vi "ExCircularBufBin2x.vi"() -> ()   [LabVIEW 2010]
panel:
  in  "Software Accumulation":u32=1 min=1 step=1
  in  "Intensifier":bool
  in  "Temperature":dbl=-10.0 format="%.2f"
  in  "Exposure":dbl min=0.0 step=1e-06 format="%.5f"
  in  "stop":bool
  in  "Store":bool
  out "error out":errorcluster
  in  "error in (no error)":errorcluster
  # "ExCircularBufBin2x:\nThis example only works with cameras with circualar buffer capability. This routine will continously display an image binned by 2 in both the x and the y direction. It will store in append mode the frames while the store toggle switch is on."
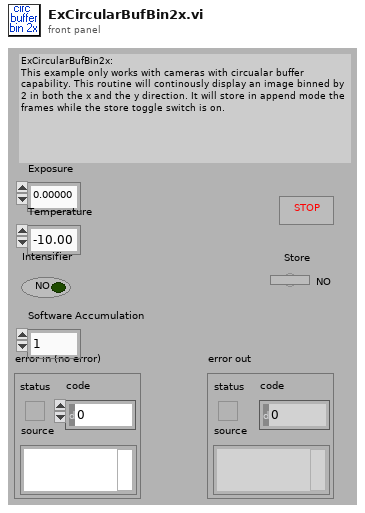
[diagram p1: front panel]
types:
  T1 = cluster{"acquire focus mode":u32, "Exposure":dbl, "Number of Images":u32, "Software Accumulation":u32}
  T2 = cluster{"Camera Handle":u32, "Pulser Handle":u32, "File Handle":u32, "Display Handle":u32, "Image Handle":u32}
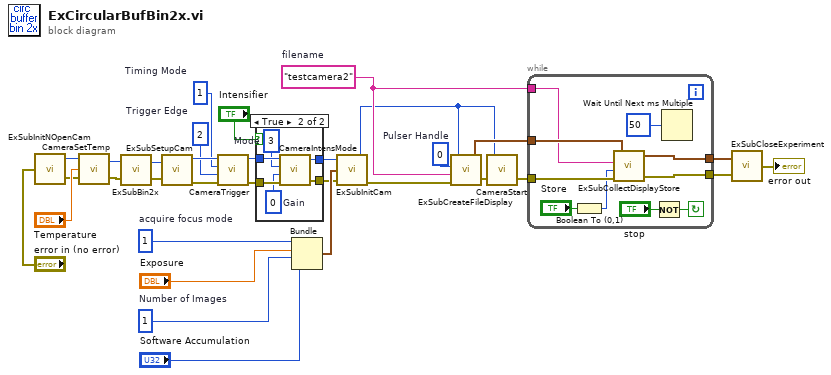
[diagram p0: block diagram]
diagram:
  w14 = u32 0  # Pulser Handle
  w15 = u32 1  # Timing Mode
  w16 = u32 2  # Trigger Edge
  w18 = u32 1  # acquire focus mode
  w17 = u32 1  # Number of Images
  w32 = "testcamera2"  # filename
  n1 = call "ExSubInitNOpenCam.vi"("error in (no error)"="error in (no error)") -> ("Camera Handle"=w4:u32, "error out"=w2:errorcluster)
  n2 = call <userlib>:"CameraSetTemp.vi"("error in (no error)"=w2, "Temperature"="Temperature", "Camera Handle"=w4) -> ("error out"=w6:errorcluster, "Camera Handle"=w5:u32)
  n3 = call "ExSubBin2x.vi"("error in (no error)"=w6, "Camera Handle"=w5) -> ("error out"=w1:errorcluster, "Camera Handle"=w19:u32)
  n4 = call "ExSubSetupCam.vi"("error in (no error)"=w1, "Camera Handle"=w19) -> ("error out"=w22:errorcluster, "Camera Handle"=w23:u32)
  n5 = call <userlib>:"CameraTrigger.vi"("error in"=w22, "Trigger Edge"=w16, "Timing Mode"=w15, "Camera Handle"=w23) -> ("error out"=w10:errorcluster, "Camera Handle"=w12:u32)
  n6 = case shown="True" "Intensifier" {
    tunnel: w12 -> [w34 w40]
    tunnel: [w34 w39] -> w11
    tunnel: w10 -> [w33 w38]
    tunnel: [w33 w37] -> w9
    frame False {
    }
    frame True {
      w35 = u32 0  # Gain
      w36 = u32 3  # Mode
      n7 = call <userlib>:"CameraIntensMode.vi"("error in"=w38, "Intensifier Gain"=w35, "Mode"=w36, "Camera Handle"=w40) -> ("error out"=w37:errorcluster, "Camera Handle"=w39:u32)
    }
  }
  n8 = Bundle("acquire focus mode"=w18, "Exposure"="Exposure", "Number of Images"=w17, "Software Accumulation"="Software Accumulation") -> (w29:T1)  [unwired: 1 in]
  n9 = call "ExSubInitCam.vi"("error in (no error)"=w9, "Camera Information"=w29, "Camera Handle"=w11) -> ("error out"=w28:errorcluster, "Camera Handle"=w13:u32)
  n10 = call "ExSubCreateFileDisplay.vi"("error in (no error)"=w28, "File and Display Name"=w32, "Pulser Handle"=w14, "Camera Handle"=w13) -> ("error out"=w20:errorcluster, "Handles Out"=w27:T2)
  n11 = call <userlib>:"CameraStart.vi"("error in"=w20, "Camera Handle"=w13) -> ("error out"=w21:errorcluster)  [unwired: 1 out]
  n12 = while {
    tunnel: w27 -> [w49]
    tunnel: w21 -> [w48]
    tunnel: w32 -> [w41]
    tunnel: [w46] -> w25
    tunnel: [w47] -> w26
    stop <- w44 continue-if-true
    n13 = Boolean To (0,1)(Boolean="Store") -> (0, 1=w42:i16)
    n14 = call "ExSubCollectDisplayStore.vi"("error in (no error)"=w48, "Store flag"=w42, "Display Title"=w41, "Handle Cluster"=w49) -> ("error out"=w46:errorcluster, "Handle Cluster Out"=w47:T2)  [unwired: 1 out]
    n15 = Not(x="stop") -> (.not. x?=w44:bool)
    n16 = Wait Until Next ms Multiple(millisecond multiple=u32 50) -> ()  [unwired: 1 out]
  }
  n17 = call "ExSubCloseExperiment.vi"("error in (no error)"=w25, "Handles In"=w26) -> ("error out"=→"error out":errorcluster)
